vi "ir test.vi"() -> ()   [LabVIEW 2012, in "BlockParty4150.lvrbt"]
uses:
  BlockParty4150.lvrbt
  <vilib>/NXT/HiTechnic/HiTechnic Controls/HiTechnic Port.ctl
  <vilib>/NXT/Block Support/NXT_InputPort.ctl
  <vilib>/NXT/HiTechnic/HiTechnic Read/HiTechnic IRSeeker Sensor_AC all.vi
  <vilib>/NXT/Dual Mode Library/Display/drawNumber.vi
panel:
  in  "stop":bool
  out "Signal Strength (Array)":u8[](array[numeric])
  out "Direction (0-9)":i16
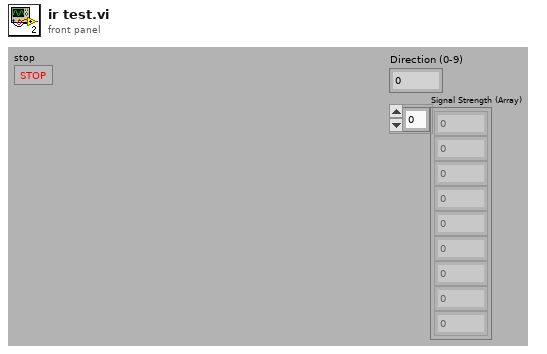
[diagram p1: front panel]
types:
  T1 = typedef "HiTechnic Port.ctl" = cluster{"Port":T2, "MUX Port":u8}
  T2 = typedef "NXT_InputPort.ctl" = u8
  T3 = cluster{"Direction (0-9)":i16, "Signal Strength (Array)":u8[]}
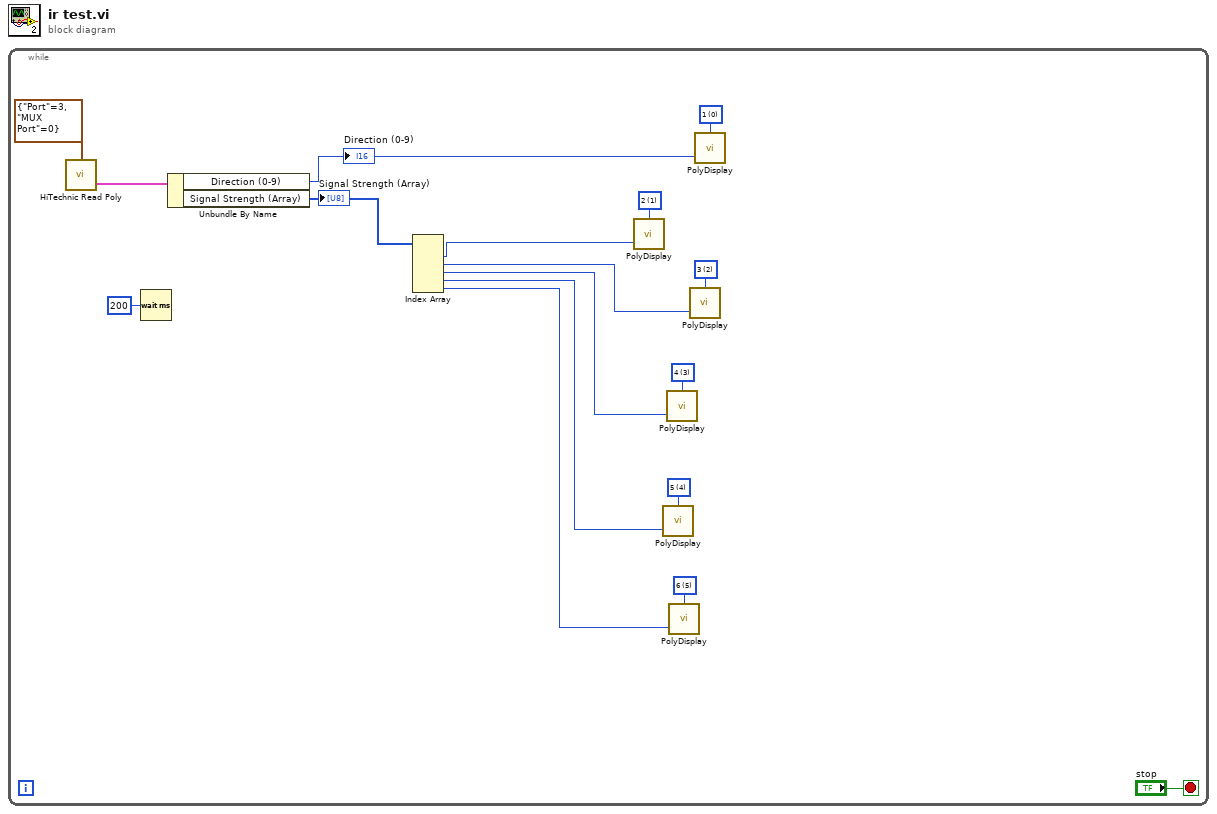
[diagram p0: block diagram]
diagram:
  n1 = while {
    stop <- "stop" stop-if-true
    w7 = i16 5 items=["1", "2", "3", "4", "5", "6", "7", "8"] ("Line")
    w8 = i16 4 items=["1", "2", "3", "4", "5", "6", "7", "8"] ("Line")
    w9 = i16 2 items=["1", "2", "3", "4", "5", "6", "7", "8"] ("Line")
    w10 = i16 1 items=["1", "2", "3", "4", "5", "6", "7", "8"] ("Line")
    w11 = i16 3 items=["1", "2", "3", "4", "5", "6", "7", "8"] ("Line")
    w12 = i16 0 items=["1", "2", "3", "4", "5", "6", "7", "8"] ("Line")
    n2 = call-poly <vilib>:"HiTechnic Read Poly.vi"("Port/MUX"=T1 {"Port"=3, "MUX Port"=0}) -> ("All Info"=w17:T3)  [unwired: 2 in, 1 out]
    n3 = Wait (ms)(milliseconds to wait=u32 200) -> ()  [unwired: 1 out]
    n4 = Unbundle By Name(w17) -> ("Direction (0-9)"=w14:i16, "Signal Strength (Array)"=w13:u8[])
    "Direction (0-9)" <- w14
    "Signal Strength (Array)" <- w13
    n5 = Index Array(array=w13) -> (element #1=w6:u8, element #2=w5:u8, element #3=w4:u8, element #4=w3:u8, element #5=w2:u8)  [unwired: 5 in]
    n6 = call-poly <vilib>:"PolyDisplay.vi"("number"=w6, "Line"=w10) -> ()  [unwired: 2 in, 1 out]
    n7 = call-poly <vilib>:"PolyDisplay.vi"("number"=w3, "Line"=w8) -> ()  [unwired: 2 in, 1 out]
    n8 = call-poly <vilib>:"PolyDisplay.vi"("number"=w4, "Line"=w11) -> ()  [unwired: 2 in, 1 out]
    n9 = call-poly <vilib>:"PolyDisplay.vi"("number"=w2, "Line"=w7) -> ()  [unwired: 2 in, 1 out]
    n10 = call-poly <vilib>:"PolyDisplay.vi"("number"=w5, "Line"=w9) -> ()  [unwired: 2 in, 1 out]
    n11 = call-poly <vilib>:"PolyDisplay.vi"("number"=w14, "Line"=w12) -> ()  [unwired: 2 in, 1 out]
  }
